vi "test_common_parent.vi"() -> ()   [LabVIEW 2021]
uses:
  CAAA/CAAA.lvclass
  CParent.lvclass
  IAAA/IAAA.lvclass
  IBar/IBar.lvclass
panel:
  out "Array 2":string[](array[string])
  out "Array":string[](array[string])
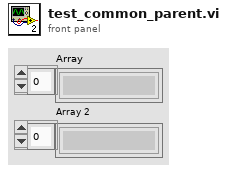
[diagram p1: front panel]
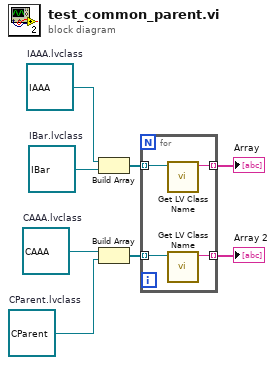
[diagram p0: block diagram]
diagram:
  w1 = refnum<class "IBar.lvclass"> refnum  # IBar.lvclass
  w5 = refnum<class "IAAA.lvclass"> refnum  # IAAA.lvclass
  w7 = refnum<class "CParent.lvclass"> refnum  # CParent.lvclass
  w8 = refnum<class "CAAA.lvclass"> refnum  # CAAA.lvclass
  n1 = Build Array(w5, w1) -> (w4:refnum<class>[])
  n2 = Build Array(w8, w7) -> (w6:refnum<class>[])
  n3 = for {
    tunnel: w6 -> [w11] mode=indexing
    tunnel: w4 -> [w12] mode=indexing
    tunnel: [w10] -> w2 mode=indexing
    tunnel: [w9] -> w3 mode=indexing
    n4 = call <vilib>:"Get LV Class Name.vi"("object"=w12) -> ("class name"=w9:string)  [unwired: 9 in, 1 out]
    n5 = call <vilib>:"Get LV Class Name.vi"("object"=w11) -> ("class name"=w10:string)  [unwired: 9 in, 1 out]
  }
  "Array" <- w3
  "Array 2" <- w2
